vi "Manipulate_TDMS_files.vi"() -> ()   [LabVIEW 2015]
panel:
  out "Adding":bool
  out "Deleting":bool
  out "name2":string
  out "name 1":string
  in  "Add Button":bool
  in  "Open Button 2":bool
  in  "Listbox 2":i32[](listbox)=[9] caption="File Name"
  out "group names 2":string[](array[string])
  out "selected path 2":path caption="selected path"
  in  "Stop Button":bool
  in  "Remove Button":bool
  in  "Listbox":i32[](listbox)=[9] caption="File Name"
  in  "Open Button":bool
  out "group names":string[](array[string])
  out "selected path":path
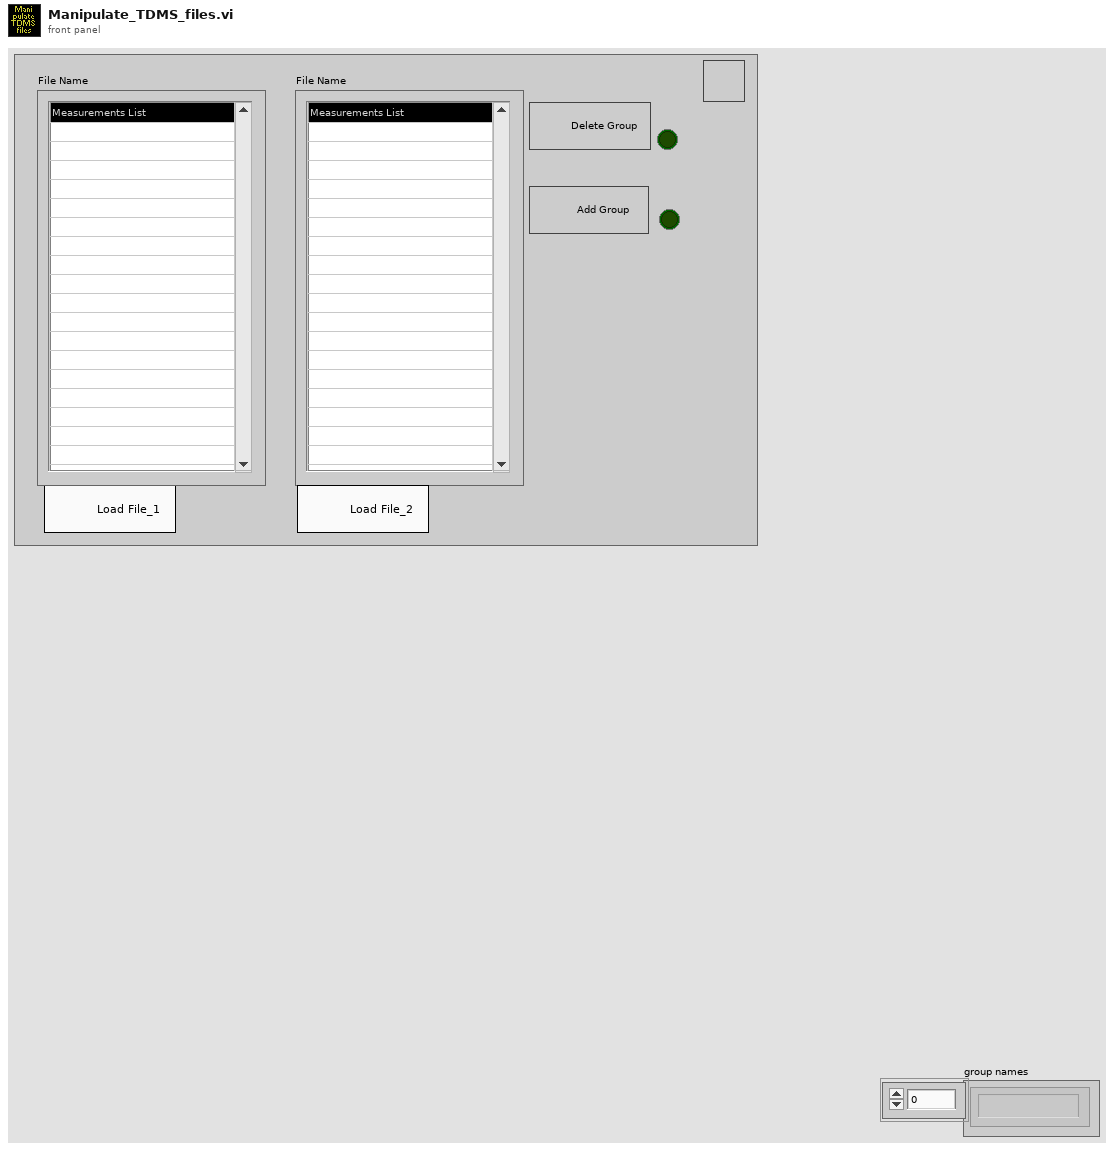
[diagram p1: front panel]
types:
  T1 = enum16{"open", "open or create", "create or replace", "create", "open (read-only)"}
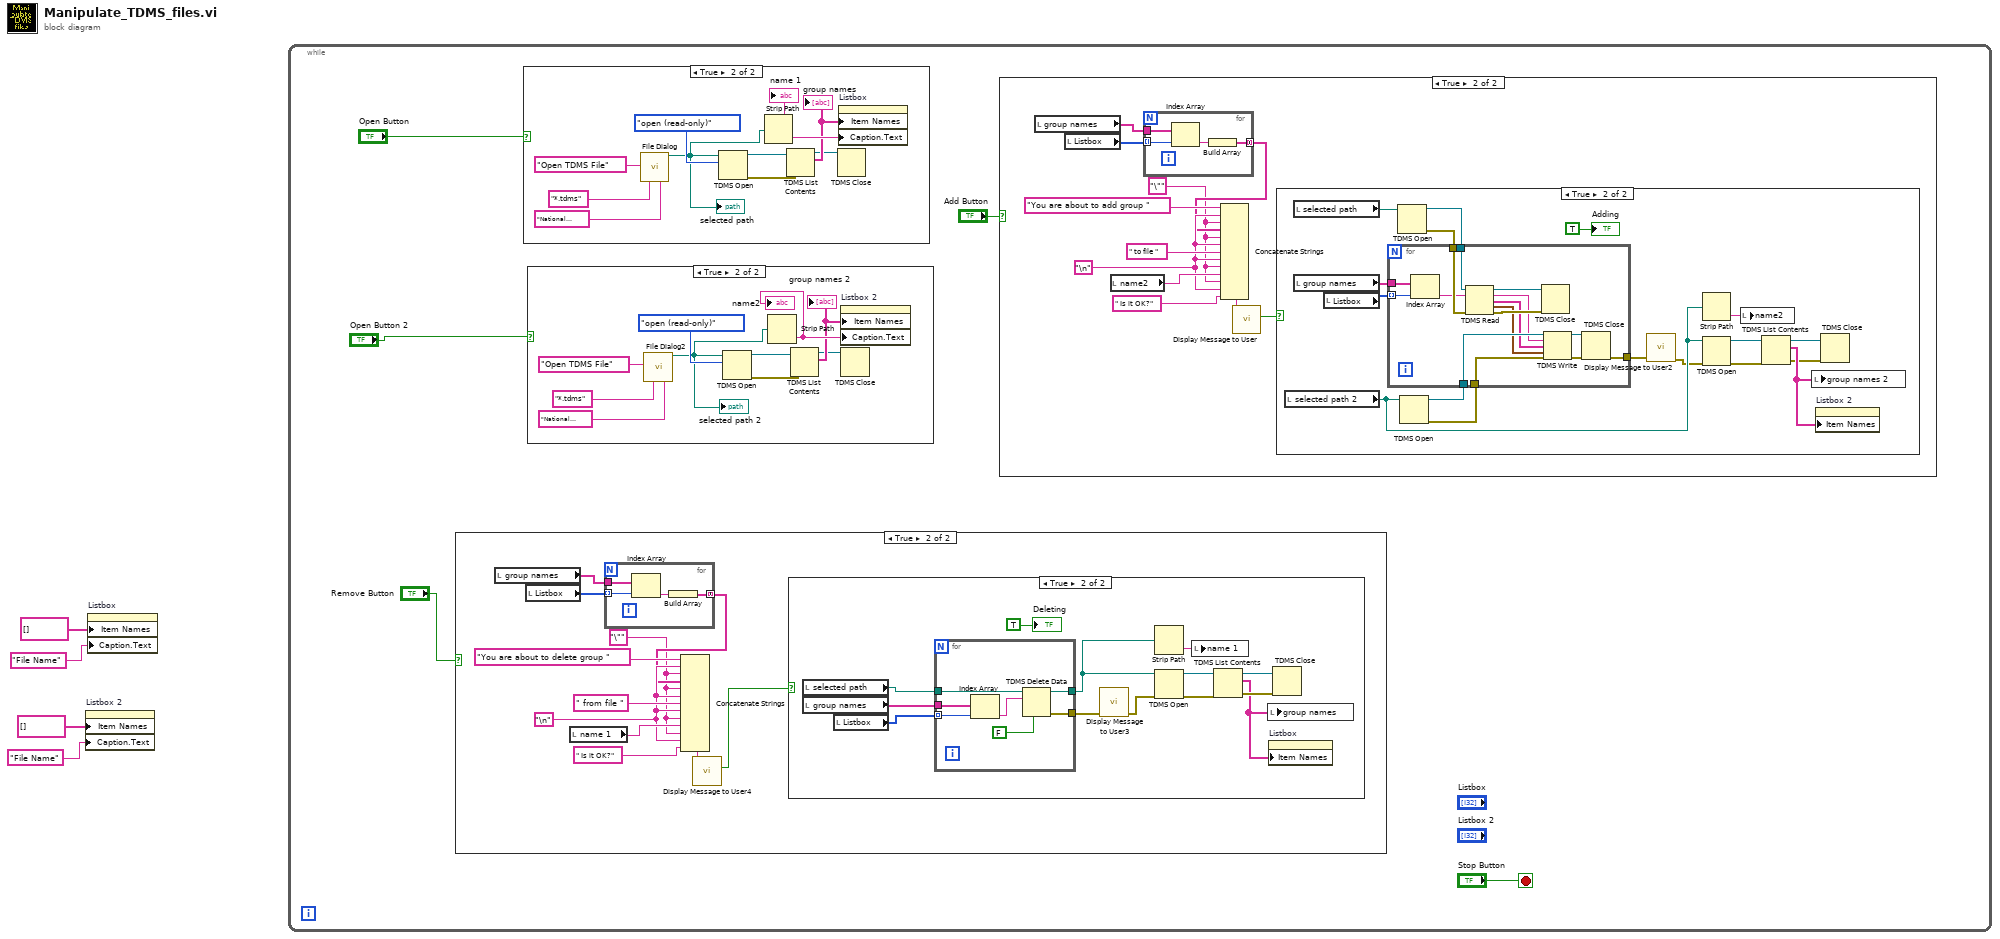
[diagram p0: block diagram]
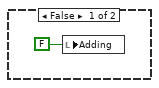
[diagram p2: hidden frame]
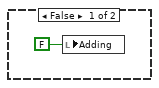
[diagram p3: hidden frame]
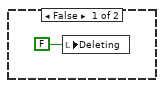
[diagram p5: hidden frame]
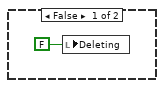
[diagram p6: hidden frame]
diagram:
  n1 = property on="Listbox 2" class="LstBox (strict)"("Item Names"=string[] [], "Caption.Text"="File Name") -> ()  [unwired: 2 in, 2 out]
  n2 = property on="Listbox" class="LstBox (strict)"("Item Names"=string[] [], "Caption.Text"="File Name") -> ()  [unwired: 2 in, 2 out]
  n3 = while {
    stop <- "Stop Button" stop-if-true
    n4 = case shown="True" "Remove Button" {
      frame False {
        n5 = local write "Deleting"(FALSE ("Deleting")) -> ()
      }
      frame True {
        w71 = "\""
        w73 = "\n"
        n6 = local read "group names"() -> (w79:string[])
        n7 = local read "Listbox"() -> (w78:i32[])
        n8 = local read "name 1"() -> (w77:string)
        n9 = for {
          tunnel: w79 -> [w84]
          tunnel: w78 -> [w83] mode=indexing
          tunnel: [w81] -> w72 mode=concatenating
          n10 = Index Array(array=w84, index=w83) -> (element=w82:string)
          n11 = Build Array(w82) -> (w81:string[])
        }
        n12 = Concatenate Strings("You are about to delete group " ("Message"), w73, w71, w72, w71, w73, " from file " ("Message"), w73, w71, w77, w71, w73, " Is it OK?" ("Message")) -> (w75:string)
        n13 = call "Display Message to User4"("Message"=w75) -> ("OK"=w70:bool)  [unwired: 9 in, 1 out]
        n14 = case shown="True" w70 {
          frame False {
            n15 = local write "Deleting"(FALSE ("Deleting")) -> ()
          }
          frame True {
            n16 = local read "selected path"() -> (w98:path)
            n17 = local read "group names"() -> (w97:string[])
            n18 = local read "Listbox"() -> (w96:i32[])
            n19 = for {
              tunnel: w98 -> [w105]
              tunnel: w97 -> [w104]
              tunnel: w96 -> [w103] mode=indexing
              tunnel: [w100] -> w95
              tunnel: [w99] -> w89
              n20 = Index Array(array=w104, index=w103) -> (element=w102:string)
              n21 = TDMS Delete Data(6:FALSE ("keep empty group/channel? (T)"), 10:w102, 11:w105) -> (0:w100:errorcluster, 3:w99:path)  [unwired: 4 in]
            }
            n22 = call "Display Message to User3"("error in (no error)"=w95) -> ("error out"=w86:errorcluster)  [unwired: 9 in, 1 out]
            n23 = Strip Path(path=w89) -> (name=w88:string)  [unwired: 1 out]
            n24 = TDMS Open(8:w86, 11:w89) -> (0:w92:errorcluster, 3:w93:refnum<k34>)  [unwired: 5 in]
            n25 = local write "name 1"(w88) -> ()
            n26 = TDMS List Contents(4:w92, 7:w93) -> (0:w90:errorcluster, 2:w87:string[], 3:w91:refnum<k34>)  [unwired: 1 in, 1 out]
            n27 = local write "group names"(w87) -> ()
            n28 = property on="Listbox" class="LstBox (strict)"("Item Names"=w87) -> ()  [unwired: 2 in, 2 out]
            n29 = TDMS Close(8:w90, 11:w91) -> ()  [unwired: 2 out]
            "Deleting" <- TRUE ("Deleting")
          }
        }
      }
    }
    n30 = case shown="True" "Open Button" {
      frame False {
      }
      frame True {
        n31 = call "File Dialog"("prompt"="Open TDMS File" ("prompt tdms"), "pattern (all files)"="*.tdms", "pattern label"="National Instruments TDM Streaming" ("pattern label tdms")) -> ("selected path"=w111:path)  [unwired: 4 in, 8 out]
        "selected path" <- w111
        n32 = TDMS Open(10:T1."open (read-only)" ("operation (0:open)"), 11:w111) -> (0:w107:errorcluster, 3:w108:refnum<k34>)  [unwired: 5 in]
        n33 = Strip Path(path=w111) -> (name=w110:string)  [unwired: 1 out]
        "name 1" <- w110
        n34 = TDMS List Contents(4:w107, 7:w108) -> (2:w109:string[], 3:w106:refnum<k34>)  [unwired: 1 in, 2 out]
        "group names" <- w109
        n35 = TDMS Close(11:w106) -> ()  [unwired: 1 in, 2 out]
        n36 = property on="Listbox" class="LstBox (strict)"("Item Names"=w109, "Caption.Text"=w110) -> ()  [unwired: 2 in, 2 out]
      }
    }
    n37 = case shown="True" "Open Button 2" {
      frame False {
      }
      frame True {
        n38 = call "File Dialog2"("prompt"="Open TDMS File" ("prompt tdms"), "pattern (all files)"="*.tdms", "pattern label"="National Instruments TDM Streaming" ("pattern label tdms")) -> ("selected path"=w64:path)  [unwired: 4 in, 8 out]
        "selected path 2" <- w64
        n39 = TDMS Open(10:T1."open (read-only)" ("operation (0:open)"), 11:w64) -> (0:w60:errorcluster, 3:w61:refnum<k34>)  [unwired: 5 in]
        n40 = Strip Path(path=w64) -> (name=w63:string)  [unwired: 1 out]
        "name2" <- w63
        n41 = TDMS List Contents(4:w60, 7:w61) -> (2:w62:string[], 3:w59:refnum<k34>)  [unwired: 1 in, 2 out]
        "group names 2" <- w62
        n42 = property on="Listbox 2" class="LstBox (strict)"("Item Names"=w62, "Caption.Text"=w63) -> ()  [unwired: 2 in, 2 out]
        n43 = TDMS Close(11:w59) -> ()  [unwired: 1 in, 2 out]
      }
    }
    n44 = case shown="True" "Add Button" {
      frame False {
        n45 = local write "Adding"(FALSE ("Adding")) -> ()
      }
      frame True {
        w11 = "\""
        w13 = "\n"
        n46 = local read "group names"() -> (w19:string[])
        n47 = local read "Listbox"() -> (w18:i32[])
        n48 = local read "name2"() -> (w17:string)
        n49 = for {
          tunnel: w19 -> [w25]
          tunnel: w18 -> [w24] mode=indexing
          tunnel: [w22] -> w12 mode=concatenating
          n50 = Index Array(array=w25, index=w24) -> (element=w23:string)
          n51 = Build Array(w23) -> (w22:string[])
        }
        n52 = Concatenate Strings("You are about to add group " ("Message"), w13, w11, w12, w11, w13, " to file " ("Message"), w13, w11, w17, w11, w13, " Is it OK?" ("Message")) -> (w15:string)
        n53 = call "Display Message to User"("Message"=w15) -> ("OK"=w21:bool)  [unwired: 9 in, 1 out]
        n54 = case shown="True" w21 {
          frame False {
            n55 = local write "Adding"(FALSE ("Adding")) -> ()
          }
          frame True {
            n56 = local read "selected path 2"() -> (w28:path)
            n57 = local read "selected path"() -> (w43:path)
            n58 = local read "group names"() -> (w42:string[])
            n59 = local read "Listbox"() -> (w41:i32[])
            n60 = TDMS Open(11:w43) -> (0:w39:errorcluster, 3:w40:refnum<k34>)  [unwired: 6 in]
            n61 = TDMS Open(11:w28) -> (0:w37:errorcluster, 3:w38:refnum<k34>)  [unwired: 6 in]
            n62 = for {
              tunnel: w42 -> [w58]
              tunnel: w41 -> [w57] mode=indexing
              tunnel: w40 -> [w56]
              tunnel: w39 -> [w55]
              tunnel: w38 -> [w51]
              tunnel: w37 -> [w50]
              tunnel: [w44] -> w36
              n63 = Index Array(array=w58, index=w57) -> (element=w54:string)
              n64 = TDMS Read(0:w56, 5:w54, 11:w55) -> (4:w53:refnum<k34>, 6:w49:string, 8:w48:string[], 10:w47:waveform(dbl)[], 15:w52:errorcluster)  [unwired: 5 in, 1 out]
              n65 = TDMS Close(8:w52, 11:w53) -> ()  [unwired: 2 out]
              n66 = TDMS Write(0:w51, 5:w49, 7:w48, 9:w47, 11:w50) -> (4:w46:refnum<k34>, 15:w45:errorcluster)  [unwired: 1 in, 2 out]
              n67 = TDMS Close(8:w45, 11:w46) -> (0:w44:errorcluster)  [unwired: 1 out]
            }
            n68 = call "Display Message to User2"("error in (no error)"=w36) -> ("error out"=w27:errorcluster)  [unwired: 9 in, 1 out]
            n69 = Strip Path(path=w28) -> (name=w33:string)  [unwired: 1 out]
            n70 = TDMS Open(8:w27, 11:w28) -> (0:w30:errorcluster, 3:w29:refnum<k34>)  [unwired: 5 in]
            n71 = local write "name2"(w33) -> ()
            n72 = TDMS List Contents(4:w30, 7:w29) -> (0:w32:errorcluster, 2:w34:string[], 3:w31:refnum<k34>)  [unwired: 1 in, 1 out]
            n73 = local write "group names 2"(w34) -> ()
            n74 = property on="Listbox 2" class="LstBox (strict)"("Item Names"=w34) -> ()  [unwired: 2 in, 2 out]
            n75 = TDMS Close(8:w32, 11:w31) -> ()  [unwired: 2 out]
            "Adding" <- TRUE ("Adding")
          }
        }
      }
    }
  }
